vi "Macro Processor.vi"(8 "error in (no error)":errorcluster, 9 "Data":variant, 10 "Argument":string, 11 "State Data":T1={"Core"={"Current VI Reference"=refnum, "Close Panel on Exit?"=FALSE}, "Macro"={"New"=refnum, "Saved"=refnum}, "Step"=0, "i_Macro"=0, "Keyboard"=refnum, "Macro Active?"=FALSE, "Macro Names"=[], "i_Step"=0, "Refs"={"Name"=refnum, "Description"=refnum, "Start"=refnum, "Steps"=refnum, "Add Step 2"=refnum, "Dbl Click"=refnum, "Start Step"=refnum, "Stop Step"=refnum, "Add Step"=refnum, "Insert Before"=refnum, "Insert After"=refnum, "Modify Step"=refnum, "Delete Step"=refnum, "Clear Steps"=refnum, "Repeat"=refnum}, "Resolutions"=[], "App Data Dir"=path "", "Start Time"=timestamp(0 s since 1904-01-01), "Results"=[], "Last Result"={"Step"="", "Actual Value"=variant, "Abort?"=FALSE, "Outcome"=enum."Skipped", "Error"={"status"=FALSE, "code"=0, "source"=""}}, "Config Path"=path "", "Config"={"Save Report?"=FALSE, "Report Path"=path "", "Macro Directory"=path "", "Macro Hotkey"=[], "Abort Hotkey"=[], "App Instances"=[]}, "Clicked Row"=0, "Start Step"=0, "Stop Step"=0, "VI-S Configured?"=FALSE}) -> (0 "error out":errorcluster, 1 "States at Back":string, 2 "States at Front":string, 3 "State Data out":T1={"Core"={"Current VI Reference"=refnum, "Close Panel on Exit?"=FALSE}, "Macro"={"New"=refnum, "Saved"=refnum}, "Step"=0, "i_Macro"=0, "Keyboard"=refnum, "Macro Active?"=FALSE, "Macro Names"=[], "i_Step"=0, "Refs"={"Name"=refnum, "Description"=refnum, "Start"=refnum, "Steps"=refnum, "Add Step 2"=refnum, "Dbl Click"=refnum, "Start Step"=refnum, "Stop Step"=refnum, "Add Step"=refnum, "Insert Before"=refnum, "Insert After"=refnum, "Modify Step"=refnum, "Delete Step"=refnum, "Clear Steps"=refnum, "Repeat"=refnum}, "Resolutions"=[], "App Data Dir"=path "", "Start Time"=timestamp(0 s since 1904-01-01), "Results"=[], "Last Result"={"Step"="", "Actual Value"=variant, "Abort?"=FALSE, "Outcome"=enum."Skipped", "Error"={"status"=FALSE, "code"=0, "source"=""}}, "Config Path"=path "", "Config"={"Save Report?"=FALSE, "Report Path"=path "", "Macro Directory"=path "", "Macro Hotkey"=[], "Abort Hotkey"=[], "App Instances"=[]}, "Clicked Row"=0, "Start Step"=0, "Stop Step"=0, "VI-S Configured?"=FALSE})   [LabVIEW 2020, in "MacroAssert.lvlib"]
doc: "Processes next states of a macro and updates relevant state data based on the current <B>State Data</B>."
uses:
  MacroAssert.lvlib
  Classes/Macro/Macro.lvclass
  Classes/Step/Step.lvclass
  Custom Errors/Custom Errors.lvlib
  CTLs/Outcome.ctl
  CTLs/Refs.ctl
  CTLs/Result.ctl
  CTLs/Config.ctl
  CTLs/State Data.ctl
  CTLs/App Instance.ctl
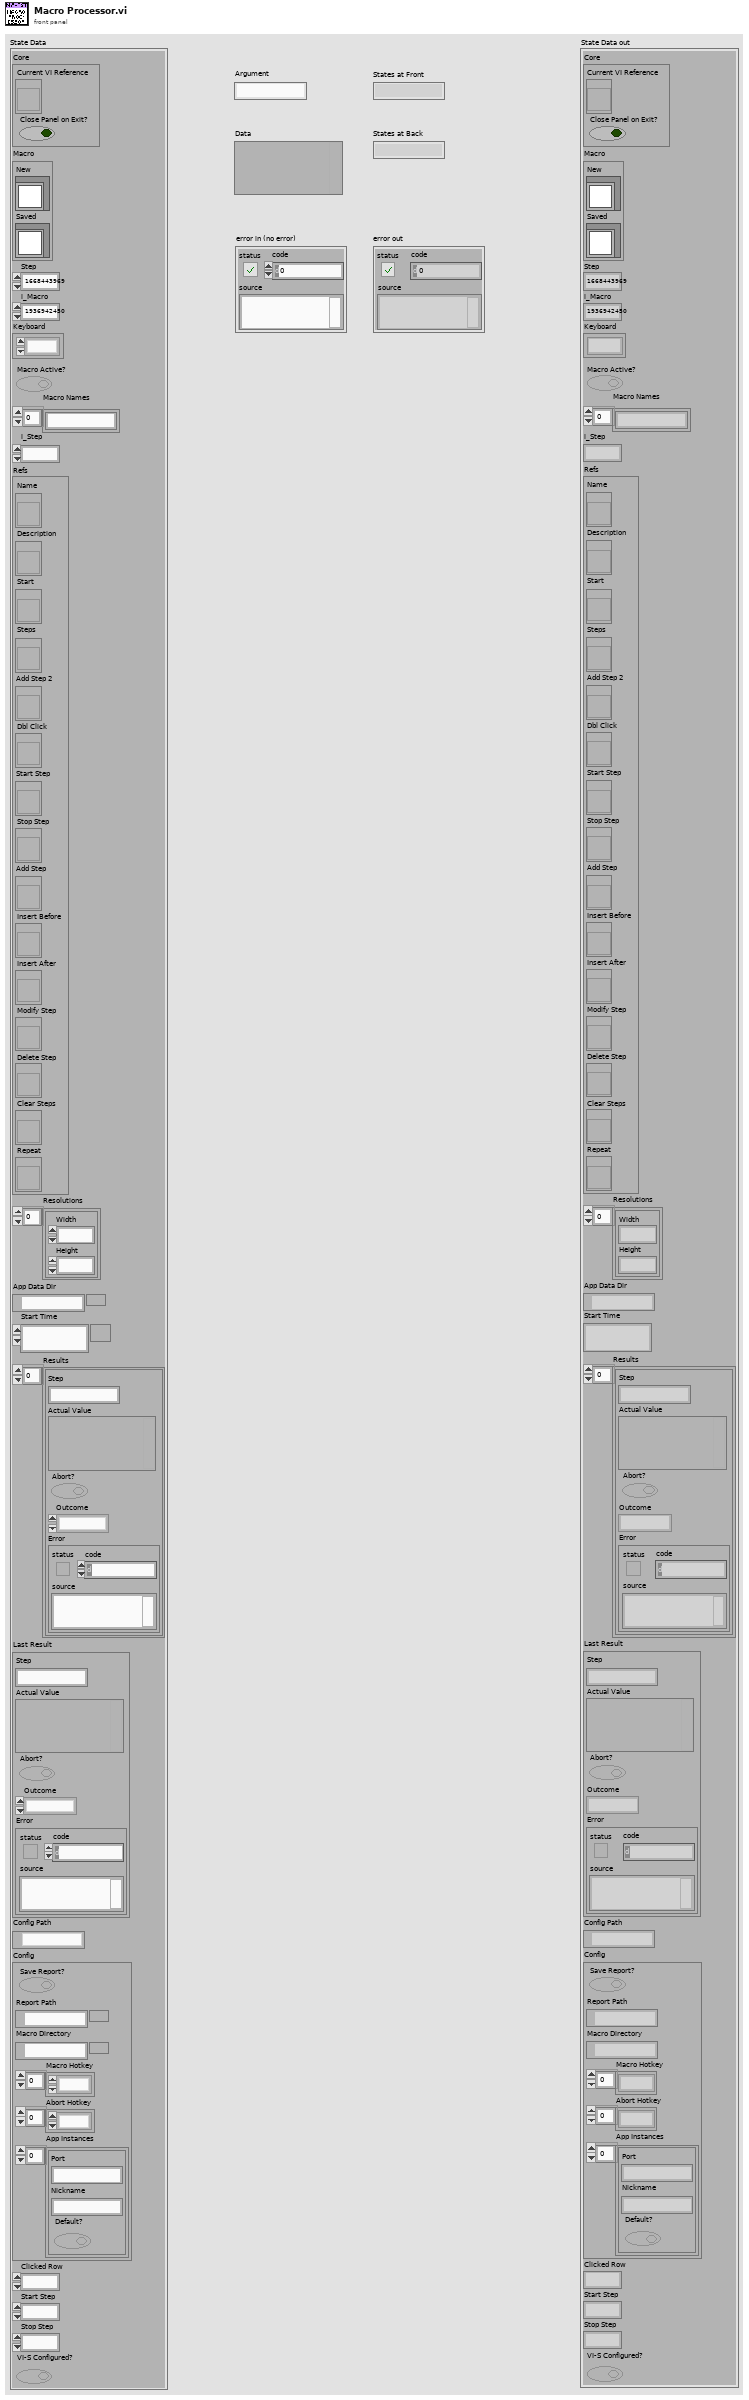
[diagram p1: front panel]
types:
  T1 = typedef "MacroAssert.lvlib/State Data.ctl" = cluster{"Core":cluster{"Current VI Reference":refnum<vi>, "Close Panel on Exit?":bool}, "Macro":cluster{"New":refnum<class "Macro.lvclass">, "Saved":refnum<class "Macro.lvclass">}, "Step":i32, "i_Macro":i32, "Keyboard":refnum<k1>, "Macro Active?":bool, "Macro Names":string[], "i_Step":i32, "Refs":T2, "Resolutions":cluster{"Width":i16, "Height":i16}[], "App Data Dir":path, "Start Time":timestamp, "Results":T3[], "Last Result":T3, "Config Path":path, "Config":T5, "Clicked Row":i32, "Start Step":i32, "Stop Step":i32, "VI-S Configured?":bool}
  T2 = typedef "MacroAssert.lvlib/Refs.ctl" = cluster{"Name":refnum<vi>, "Description":refnum<vi>, "Start":refnum<vi>, "Steps":refnum<vi>, "Add Step 2":refnum<vi>, "Dbl Click":refnum<vi>, "Start Step":refnum<vi>, "Stop Step":refnum<vi>, "Add Step":refnum<vi>, "Insert Before":refnum<vi>, "Insert After":refnum<vi>, "Modify Step":refnum<vi>, "Delete Step":refnum<vi>, "Clear Steps":refnum<vi>, "Repeat":refnum<vi>}
  T3 = typedef "MacroAssert.lvlib/Result.ctl" = cluster{"Step":string, "Actual Value":variant, "Abort?":bool, "Outcome":T4, "Error":errorcluster}
  T4 = typedef "MacroAssert.lvlib/Outcome.ctl" = enum16{"Not Started", "Skipped", "Pass", "Fail", "Complete", "Error", "Auto Abort", "User Abort"}
  T5 = typedef "MacroAssert.lvlib/Config.ctl" = cluster{"Save Report?":bool, "Report Path":path, "Macro Directory":path, "Macro Hotkey":enum16{"0", "1", "2", "3", "4", "5", "6", "7", "8", "9", "A", "B", "C", "D", "E", "F", "G", "H", "I", "J", "K", "L", "M", "N", "O", "P", "Q", "R", "S", "T", "U", "V", "W", "X", "Y", "Z", "F1", "F2", "F3", "F4", "F5", "F6", "F7", "F8", "F9", "F10", "F11", "F12", "F13", "F14", "F15", "ADD", "BACK", "BACKSLASH", "CAPITAL", "COMMA", "DECIMAL", "DELETE", "DIVIDE", "DOWN", "END", "EQUALS", "ESCAPE", "GRAVE (`)", "HOME", "INSERT", "LBRACKET", "LCONTROL", "LEFT", "L ALT", "LSHIFT", "LWIN", "MINUS", "MULTIPLY", "NEXT", "NUMLOCK", "NUMPAD_0", "NUMPAD_1", "NUMPAD_2", "NUMPAD_3", "NUMPAD_4", "NUMPAD_5", "NUMPAD_6", "NUMPAD_7", "NUMPAD_8", "NUMPAD_9", "PAUSE", "PERIOD", "PRIOR (PG UP)", "RBRACKET", "RCONTROL", "RETURN", "RIGHT", "R ALT", "RSHIFT", "RWIN", "SCROLL", "SEMICOLON", "SLASH", "SPACE", "SUBTRACT", "TAB", "UP", "ENTER (num pad)", "' (quote)"}[], "Abort Hotkey":enum16{"0", "1", "2", "3", "4", "5", "6", "7", "8", "9", "A", "B", "C", "D", "E", "F", "G", "H", "I", "J", "K", "L", "M", "N", "O", "P", "Q", "R", "S", "T", "U", "V", "W", "X", "Y", "Z", "F1", "F2", "F3", "F4", "F5", "F6", "F7", "F8", "F9", "F10", "F11", "F12", "F13", "F14", "F15", "ADD", "BACK", "BACKSLASH", "CAPITAL", "COMMA", "DECIMAL", "DELETE", "DIVIDE", "DOWN", "END", "EQUALS", "ESCAPE", "GRAVE (`)", "HOME", "INSERT", "LBRACKET", "LCONTROL", "LEFT", "L ALT", "LSHIFT", "LWIN", "MINUS", "MULTIPLY", "NEXT", "NUMLOCK", "NUMPAD_0", "NUMPAD_1", "NUMPAD_2", "NUMPAD_3", "NUMPAD_4", "NUMPAD_5", "NUMPAD_6", "NUMPAD_7", "NUMPAD_8", "NUMPAD_9", "PAUSE", "PERIOD", "PRIOR (PG UP)", "RBRACKET", "RCONTROL", "RETURN", "RIGHT", "R ALT", "RSHIFT", "RWIN", "SCROLL", "SEMICOLON", "SLASH", "SPACE", "SUBTRACT", "TAB", "UP", "ENTER (num pad)", "' (quote)"}[], "App Instances":T6[]}
  T6 = typedef "MacroAssert.lvlib/App Instance.ctl" = cluster{"Port":string, "Nickname":string, "Default?":bool}
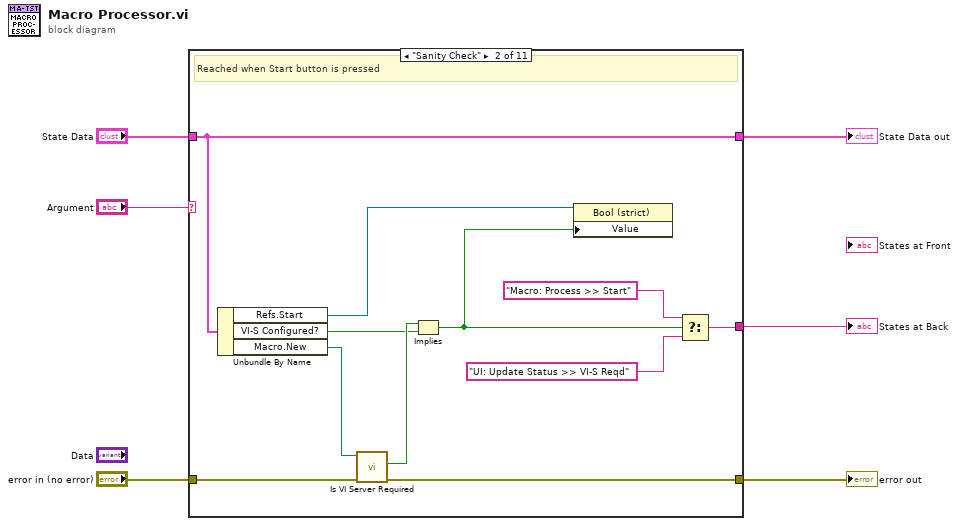
[diagram p0: block diagram]
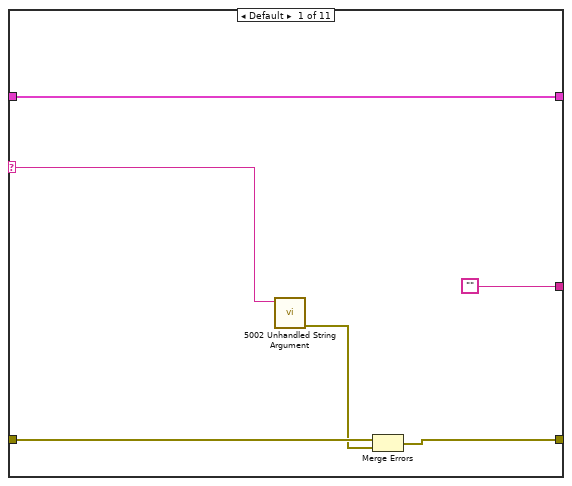
[diagram p2: hidden frame]
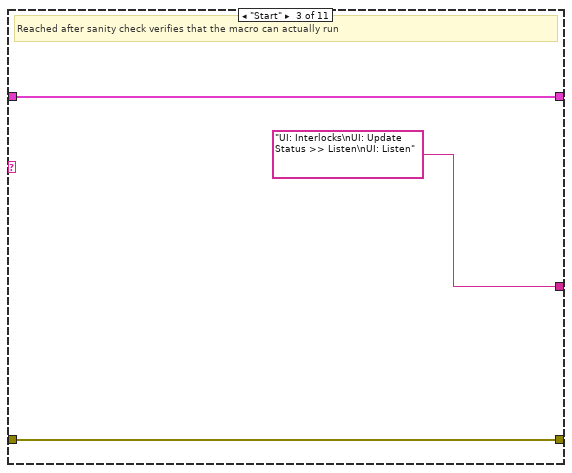
[diagram p3: hidden frame]
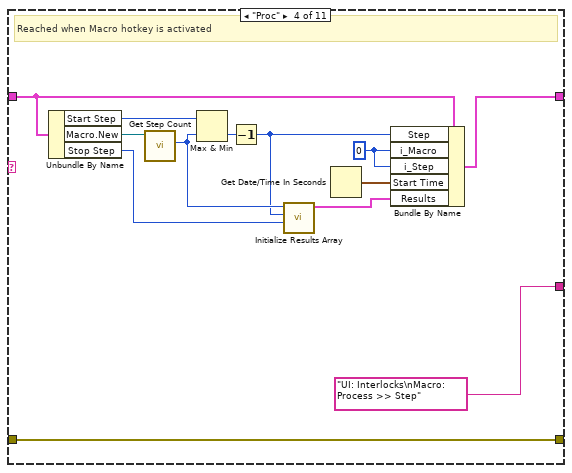
[diagram p4: hidden frame]
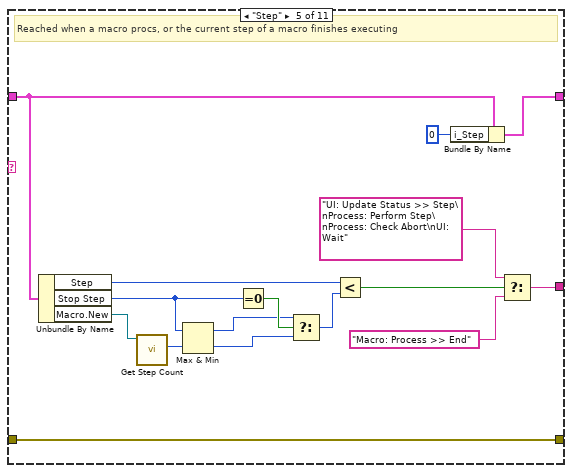
[diagram p5: hidden frame]
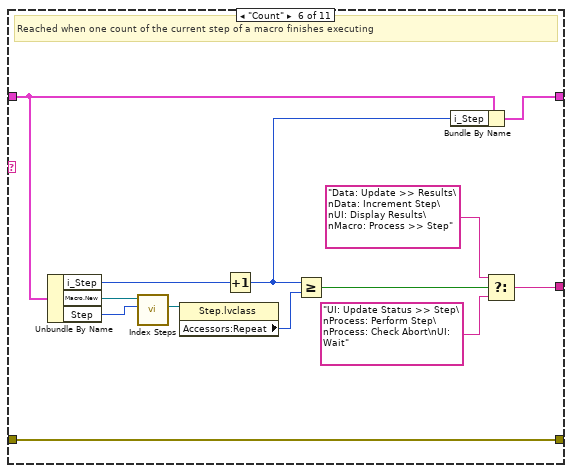
[diagram p6: hidden frame]
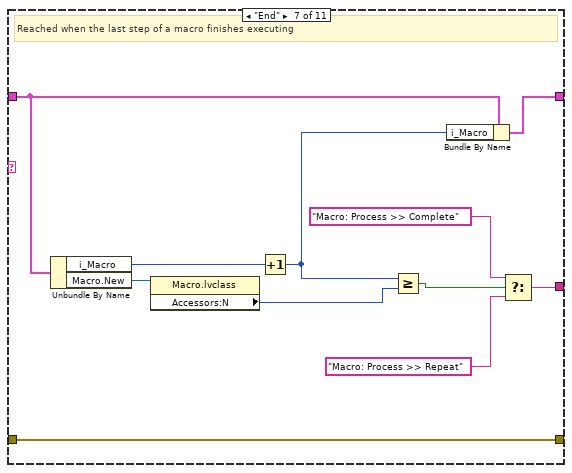
[diagram p7: hidden frame]
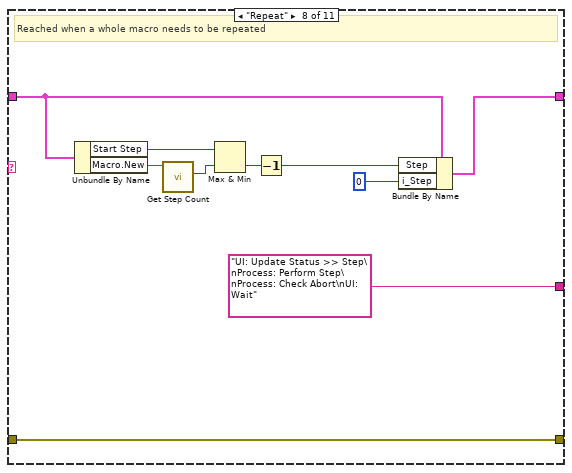
[diagram p8: hidden frame]
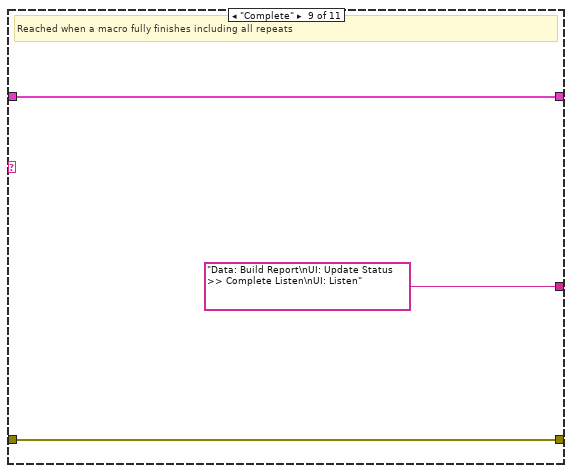
[diagram p9: hidden frame]
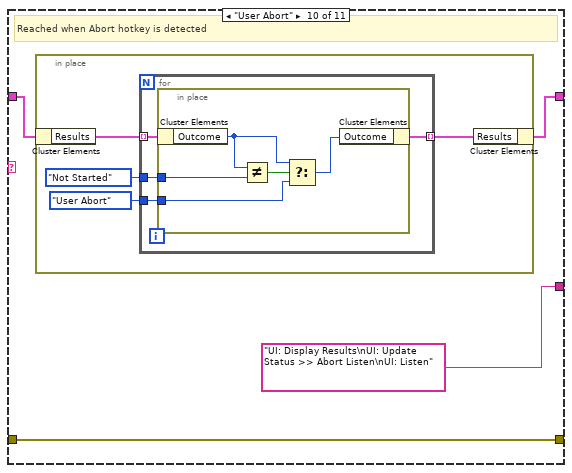
[diagram p10: hidden frame]
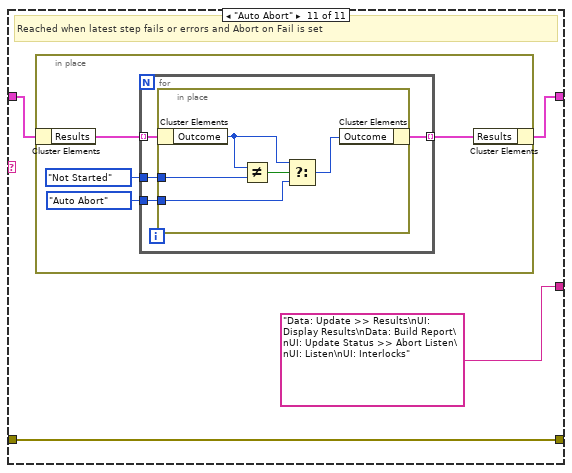
[diagram p11: hidden frame]
diagram:
  n1 = case shown="\"Sanity Check\"" "Argument" {
    selector: "Argument" -> [w9 _ _ _ _ _ _ _ _ _ _]
    tunnel: "State Data" -> [w8 w22 w25 w34 w52 w66 w77 w82 w90 w94 w111]
    tunnel: [w8 w22 w25 w39 w51 w65 w75 w89 w90 w93 w110] -> w4
    tunnel: ["" w18 "UI: Interlocks\nUI: Update Status >> Listen\nUI: Listen" "UI: Interlocks\nMacro: Process >> Step" w49 w63 w73 "UI: Update Status >> Step\nProcess: Perform Step\nProcess: Check Abort\nUI: Wait" "Data: Build Report\nUI: Update Status >> Complete Listen\nUI: Listen" "UI: Display Results\nUI: Update Status >> Abort Listen\nUI: Listen" "Data: Update >> Results\nUI: Display Results\nData: Build Report\nUI: Update Status >> Abort Listen\nUI: Listen\nUI: Interlocks"] -> w3
    tunnel: "error in (no error)" -> [w12 w23 w24 w31 w40 w57 w69 w80 w91 w95 w112]
    tunnel: [w10 w21 w24 w31 w40 w57 w69 w80 w91 w95 w112] -> w1
    frame Default {
      n2 = call "5002 Unhandled String Argument.vi"("Argument"=w9) -> ("error out"=w11:errorcluster)  [unwired: 10 in]
      n3 = Merge Errors(w12, w11) -> (w10:errorcluster)
    }
    frame "Sanity Check" {
      # "Reached when Start button is pressed"
      n4 = Unbundle By Name(w22) -> ("Refs.Start"=w15:refnum<vi>, "VI-S Configured?"=w13:bool, "Macro.New"=w14:refnum<class "Macro.lvclass">)
      n5 = call-dynamic "Is VI Server Required.vi"("error in (no error)"=w23, "Macro in"=w14) -> ("error out"=w21:errorcluster, "VI Server Required?"=w20:bool)  [unwired: 7 in, 1 out]
      n6 = Implies(1:w13, 2:w20) -> (0:w16:bool)
      n7 = property class="Bool (strict)"(reference=w15, "Value"=w16) -> ()  [unwired: 1 in, 2 out]
      n8 = Select(t="Macro: Process >> Start", s=w16, f="UI: Update Status >> VI-S Reqd") -> (s? t:f=w18:string)
    }
    frame "Start" {
      # "Reached after sanity check verifies that the macro can actually run"
    }
    frame "Proc" {
      w38 = 0 ("Step")
      # "Reached when Macro hotkey is activated"
      n9 = Unbundle By Name(w34) -> ("Start Step"=w33:i32, "Macro.New"=w35:refnum<class "Macro.lvclass">, "Stop Step"=w28:i32)
      n10 = call-dynamic "Get Step Count.vi"("Macro in"=w35) -> ("Step Count"=w30:i32)  [unwired: 8 in, 2 out]
      n11 = Max & Min(x=w33, y=w30) -> (min(x,y)=w32:i32)  [unwired: 1 out]
      n12 = Decrement(x=w32) -> (x-1=w29:i32)
      n13 = call "Initialize Results Array.vi"("Stop Step"=w28, "Start Step"=w29, "Step Count"=w30) -> ("Results"=w27:T3[])  [unwired: 8 in]
      n14 = Get Date/Time In Seconds() -> (seconds since 1Jan1904=w37:timestamp)
      n15 = Bundle By Name(cluster=w34, "Step"=w29, "i_Macro"=w38, "i_Step"=w38, "Start Time"=w37, "Results"=w27) -> (w39:T1)
    }
    frame "Step" {
      # "Reached when a macro procs, or the current step of a macro finishes executing"
      n16 = Unbundle By Name(w52) -> ("Step"=w55:i32, "Stop Step"=w45:i32, "Macro.New"=w47:refnum<class "Macro.lvclass">)
      n17 = call-dynamic "Get Step Count.vi"("Macro in"=w47) -> ("Step Count"=w46:i32)  [unwired: 8 in, 2 out]
      n18 = Max & Min(x=w45, y=w46) -> (max(x,y)=w42:i32, min(x,y)=w43:i32)
      n19 = Equal To 0?(x=w45) -> (x = 0?=w44:bool)
      n20 = Select(t=w42, s=w44, f=w43) -> (s? t:f=w41:i32)
      n21 = Less?(x=w55, y=w41) -> (x < y?=w54:bool)
      n22 = Bundle By Name(cluster=w52, "i_Step"=0 ("Rcount")) -> (w51:T1)
      n23 = Select(t="UI: Update Status >> Step\nProcess: Perform Step\nProcess: Check Abort\nUI: Wait", s=w54, f="Macro: Process >> End") -> (s? t:f=w49:string)
    }
    frame "Count" {
      # "Reached when one count of the current step of a macro finishes executing"
      n24 = Unbundle By Name(w66) -> ("i_Step"=w62:i32, "Macro.New"=w61:refnum<class "Macro.lvclass">, "Step"=w60:i32)
      n25 = call-dynamic "Index Steps.vi"("Index"=w60, "Macro in"=w61) -> ("Step"=w59:refnum<class "Step.lvclass">)  [unwired: 7 in, 2 out]
      n26 = property class="Step.lvclass"(reference=w59) -> ("Accessors:Repeat"=w58:i32)  [unwired: 1 in, 2 out]
      n27 = Increment(x=w62) -> (x+1=w56:i32)
      n28 = Greater Or Equal?(x=w56, y=w58) -> (x >= y?=w68:bool)
      n29 = Bundle By Name(cluster=w66, "i_Step"=w56) -> (w65:T1)
      n30 = Select(t="Data: Update >> Results\nData: Increment Step\nUI: Display Results\nMacro: Process >> Step", s=w68, f="UI: Update Status >> Step\nProcess: Perform Step\nProcess: Check Abort\nUI: Wait") -> (s? t:f=w63:string)
    }
    frame "End" {
      # "Reached when the last step of a macro finishes executing"
      n31 = Unbundle By Name(w77) -> ("i_Macro"=w79:i32, "Macro.New"=w71:refnum<class "Macro.lvclass">)
      n32 = property class="Macro.lvclass"(reference=w71) -> ("Accessors:N"=w70:i32)  [unwired: 1 in, 2 out]
      n33 = Increment(x=w79) -> (x+1=w76:i32)
      n34 = Greater Or Equal?(x=w76, y=w70) -> (x >= y?=w72:bool)
      n35 = Bundle By Name(cluster=w77, "i_Macro"=w76) -> (w75:T1)
      n36 = Select(t="Macro: Process >> Complete", s=w72, f="Macro: Process >> Repeat") -> (s? t:f=w73:string)
    }
    frame "Repeat" {
      # "Reached when a whole macro needs to be repeated"
      n37 = Unbundle By Name(w82) -> ("Start Step"=w84:i32, "Macro.New"=w86:refnum<class "Macro.lvclass">)
      n38 = call-dynamic "Get Step Count.vi"("Macro in"=w86) -> ("Step Count"=w85:i32)  [unwired: 8 in, 2 out]
      n39 = Max & Min(x=w84, y=w85) -> (min(x,y)=w83:i32)  [unwired: 1 out]
      n40 = Decrement(x=w83) -> (x-1=w81:i32)
      n41 = Bundle By Name(cluster=w82, "Step"=w81, "i_Step"=0 ("Step")) -> (w89:T1)
    }
    frame "Complete" {
      # "Reached when a macro fully finishes including all repeats"
    }
    frame "User Abort" {
      # "Reached when Abort hotkey is detected"
      n42 = in-place {
        n43 = in-place-cluster #1(w94) -> ("Results"=w100:T3[])
        n44 = for {
          tunnel: w100 -> [w104] mode=indexing
          tunnel: Outcome."Not Started" ("y") -> [w103]
          tunnel: [w102] -> w98 mode=indexing
          tunnel: Outcome."User Abort" ("y") -> [w101]
          n45 = in-place {
            in-place-border: w103 -> [w108]
            in-place-border: w101 -> [w105]
            n46 = in-place-cluster #2(w104) -> ("Outcome"=w107:T4)
            n47 = Not Equal?(x=w107, y=w108) -> (x != y?=w109:bool)
            n48 = Select(t=w107, s=w109, f=w105) -> (s? t:f=w106:T4)
            n49 = in-place-cluster #2("Outcome"=w106) -> (w102:T3)
          }
        }
        n50 = in-place-cluster #1("Results"=w98) -> (w93:T1)
      }
    }
    frame "Auto Abort" {
      # "Reached when latest step fails or errors and Abort on Fail is set"
      n51 = in-place {
        n52 = in-place-cluster #3(w111) -> ("Results"=w117:T3[])
        n53 = for {
          tunnel: w117 -> [w121] mode=indexing
          tunnel: Outcome."Not Started" ("y") -> [w120]
          tunnel: [w119] -> w115 mode=indexing
          tunnel: Outcome."Auto Abort" ("y") -> [w118]
          n54 = in-place {
            in-place-border: w120 -> [w125]
            in-place-border: w118 -> [w122]
            n55 = in-place-cluster #4(w121) -> ("Outcome"=w124:T4)
            n56 = Not Equal?(x=w124, y=w125) -> (x != y?=w126:bool)
            n57 = Select(t=w124, s=w126, f=w122) -> (s? t:f=w123:T4)
            n58 = in-place-cluster #4("Outcome"=w123) -> (w119:T3)
          }
        }
        n59 = in-place-cluster #3("Results"=w115) -> (w110:T1)
      }
    }
  }
  "error out" <- w1
  "State Data out" <- w4
  "States at Back" <- w3
